vi "createElement.vi"(8 "data":variant, 10 "cmdclass":string, 11 "cmd":string) -> (3 "element":T1)   [LabVIEW 2017]
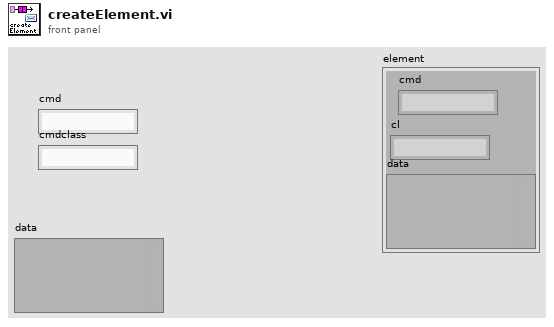
[diagram p1: front panel]
types:
  T1 = cluster{"cmd":string, "cl":string, "data":variant}
  T2 = cluster{"cmd":string, "cmdclass":string, "data":variant}
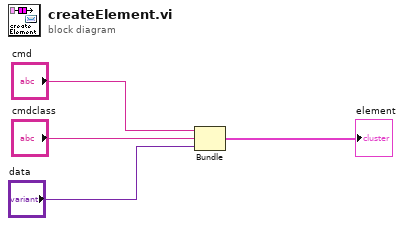
[diagram p0: block diagram]
diagram:
  n1 = Bundle("cmd"="cmd", "cmdclass"="cmdclass", "data"="data") -> (→"element":T2)  [unwired: 1 in]
